vi "Receiver.vi"(8 "ErrorArray":errorcluster[](array[cluster])) -> (0 "ErrorArray":errorcluster[](array[cluster]), 1 "XMLData":string, 2 "Command":string, 4 "error out":errorcluster, 5 "bytes_read":i32)   [LabVIEW 2017, in "Comms.lvlib"]
uses:
  Comms.lvlib
  CommsData.ctl
  <userlib>/NIST/Socket Class/Classes/Socket.TCP/Socket.TCP.lvclass
  <userlib>/NIST/NISTErrorLib/NISTErrorLib.lvlib
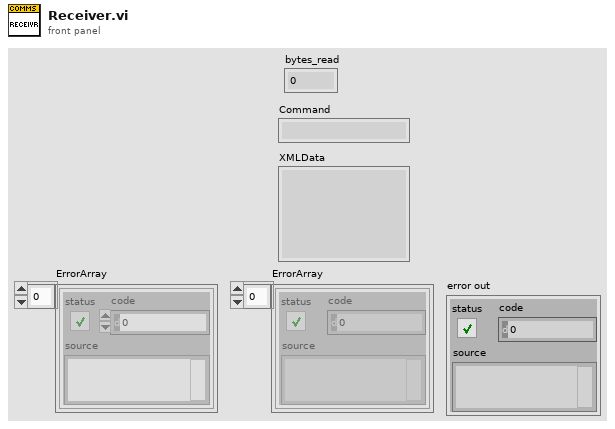
[diagram p1: front panel]
types:
  T1 = typedef "Comms.lvlib/CommsData.ctl" = cluster{"Command":string, "XMLData":string}
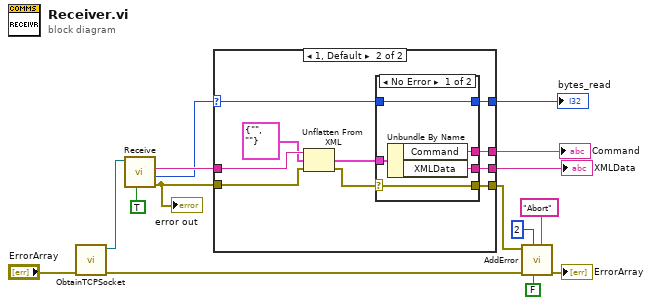
[diagram p0: block diagram]
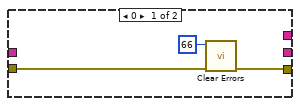
[diagram p2: hidden frame]
diagram:
  n1 = call "ObtainTCPSocket.vi"("ErrorArray"="ErrorArray") -> ("ErrorArray"=w12:errorcluster[], "SocketRef"=w13:refnum<class "Socket.TCP.lvclass">)  [unwired: 9 in]
  n2 = call-dynamic "Receive.vi"("clear_timeout_error (f)"=TRUE, "Socket.TCP in"=w13) -> ("error out"=w1:errorcluster, "bytes_read"=w7:i32, "data_out"=w11:string)  [unwired: 6 in, 1 out]
  "error out" <- w1
  n3 = case shown="1, Default" w7 {
    selector: w7 -> [_ w22]
    tunnel: w11 -> [_ w28]
    tunnel: [_ w25] -> w10
    tunnel: [_ w24] -> w9
    tunnel: [w17 w19] -> w2
    tunnel: w1 -> [w18 w23]
    tunnel: [_ w21] -> w6
    frame 0 {
      n4 = call <vilib>:"Clear Errors.vi"("error in (no error)"=w18, "specific error code to clear (0: all)"=66) -> ("error out"=w17:errorcluster)  [unwired: 4 in, 1 out]
    }
    frame 1, Default {
      n5 = Unflatten From XML(xml string=w28, type=T1 {"Command"="", "XMLData"=""} ("CommsData"), error in (no error)=w23) -> (value=w26:T1, error out=w20:errorcluster)
      n6 = case shown="No Error" w20 {
        selector: w20 -> [w29 w34]
        tunnel: w26 -> [w33 _]
        tunnel: [w32 _] -> w25
        tunnel: [w31 _] -> w24
        tunnel: w22 -> [w30 _]
        tunnel: [w30 _] -> w21
        tunnel: [w29 w34] -> w19
        frame No Error {
          n7 = Unbundle By Name(w33) -> ("Command"=w32:string, "XMLData"=w31:string)
        }
        frame Error {
        }
      }
    }
  }
  "Command" <- w10
  "XMLData" <- w9
  "bytes_read" <- w6
  n8 = call <userlib>:"AddError.vi"("Severity"="Abort", "Passthrough (f)"=FALSE, "Priority"=u8 2, "ErrorArray"=w12, "error in (no error)"=w2) -> ("ErrorArray"=→"ErrorArray":errorcluster[])  [unwired: 5 in, 1 out]
